vi "set allowedSubNode.vi"(8 "error in (no error)":errorcluster, 10 "Allowed subNode[]":string[](array[string]), 11 "xceDataNode in":refnum<class "xceDataNode.lvclass">) -> (0 "error out":errorcluster, 3 "xceDataNode out":refnum<class "xceDataNode.lvclass">)   [LabVIEW 2013, in "xceDataNode.lvclass"]
doc: "Set allowedSubNode. Filters what types of node classes are allowed to be a subNode of this class."
uses:
  xceDataNode.lvclass
  xceDataNode.lvclass/xceDataNode.ctl
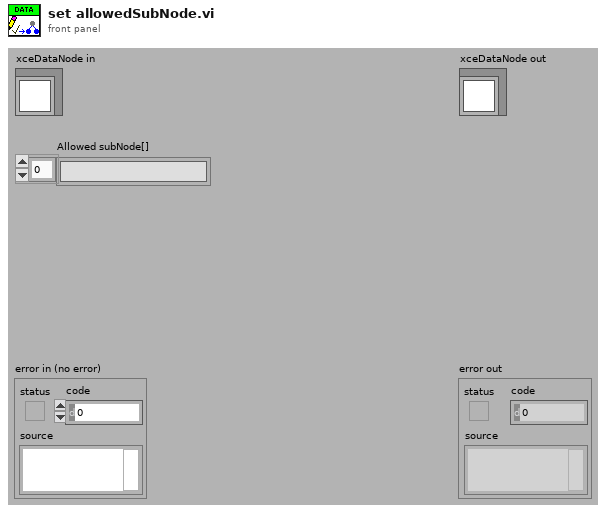
[diagram p1: front panel]
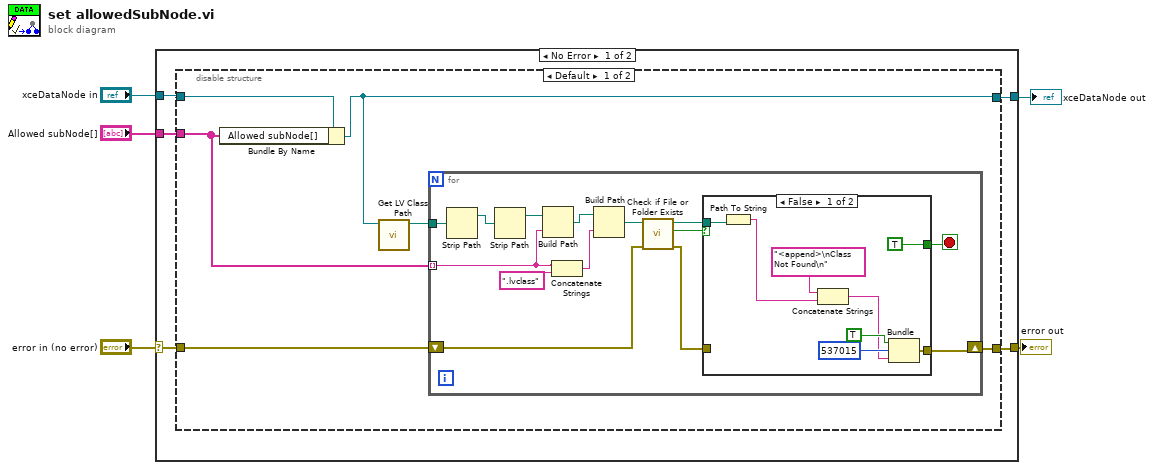
[diagram p0: block diagram]
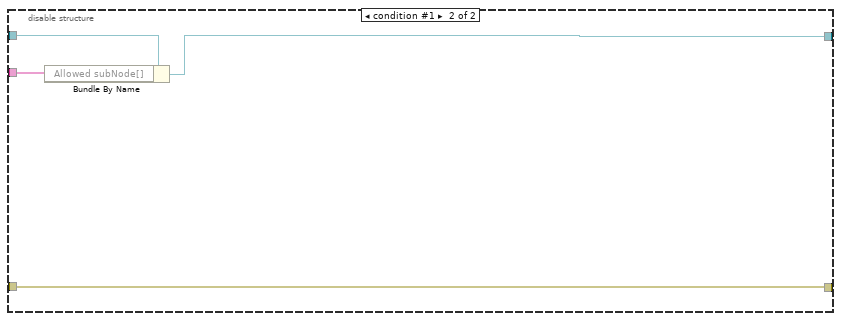
[diagram p3: hidden frame]
diagram:
  n1 = case shown="No Error" "error in (no error)" {
    selector: "error in (no error)" -> [w10 w44]
    tunnel: [w9 w44] -> w4
    tunnel: [w8 w45] -> w2
    tunnel: "xceDataNode in" -> [w6 w45]
    tunnel: "Allowed subNode[]" -> [w7 _]
    frame No Error {
      n2 = disable-structure shown="Default" {
        disable-tunnel: w7 -> [w13 w42]
        disable-tunnel: w10 -> [w16 w43]
        disable-tunnel: w6 -> [w12 w41]
        disable-tunnel: [w11 w40] -> w8
        disable-tunnel: [w15 w43] -> w9
        frame condition #0 (active) {
          n3 = Bundle By Name(cluster=w12, "Allowed subNode[]"=w13) -> (w11:refnum<class "xceDataNode.lvclass">)
          n4 = call <vilib>:"Get LV Class Path.vi"("object"=w11) -> ("class path"=w14:path)  [unwired: 9 in, 1 out]
          n5 = for {
            tunnel: w13 -> [w19] mode=indexing
            tunnel: w14 -> [w24]
            shift-right: [w27] -> w15
            shift-left: w16 -> [w30]
            stop <- w17 stop-if-true
            n6 = Strip Path(path=w24) -> (stripped path=w23:path)  [unwired: 1 out]
            n7 = Strip Path(path=w23) -> (stripped path=w22:path)  [unwired: 1 out]
            n8 = Build Path(base path=w22, name or relative path=w19) -> (appended path=w21:path)
            n9 = Concatenate Strings(w19, ".lvclass" ("string")) -> (w20:string)
            n10 = Build Path(base path=w21, name or relative path=w20) -> (appended path=w26:path)
            n11 = call <vilib>:"Check if File or Folder Exists.vi"("error in (no error)"=w30, "path"=w26) -> ("error out"=w28:errorcluster, "file or folder exists?"=w29:bool, "dup path"=w25:path)  [unwired: 7 in]
            n12 = case shown="False" w29 {
              tunnel: w28 -> [_ w39]
              tunnel: [w34 w39] -> w27
              tunnel: w25 -> [w32 _]
              tunnel: [TRUE _] -> w17
              frame False {
                n13 = Path To String(path=w32) -> (string=w33:string)
                n14 = Concatenate Strings("<append>\nClass Not Found\n" ("source"), w33) -> (w36:string)
                n15 = Bundle("status"=TRUE, "code"=537015, w36) -> (w34:cluster{"status":bool, "code":i32, string})  [unwired: 1 out]
              }
              frame True {
              }
            }
          }
        }
        frame condition #1 {
          n16 = Bundle By Name(cluster=w41, "Allowed subNode[]"=w42) -> (w40:refnum<class "xceDataNode.lvclass">)
        }
      }
    }
    frame Error {
    }
  }
  "error out" <- w4
  "xceDataNode out" <- w2
